vi "PWROpen.vi"(8 "error in (no error)":errorcluster {"code" format="%.0x"}, 11 "PWR In":refnum<visa-resource-name>) -> (0 "error out":errorcluster, 3 "PWR Out":refnum<visa-resource-name>, 5 "PWRID":u8)   [LabVIEW 2015]
uses:
  <instrlib>/Agilent N87XX Series/Agilent N87XX Series.lvlib
  <instrlib>/Agilent N6700 Series/Agilent N6700 Series.lvlib
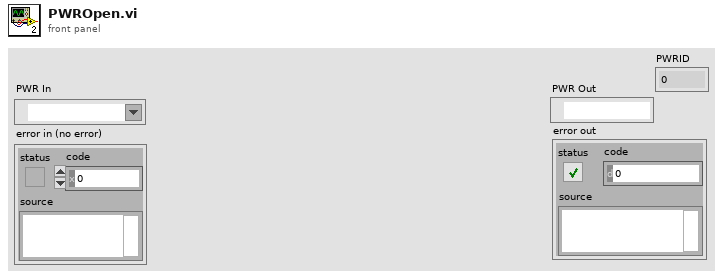
[diagram p1: front panel]
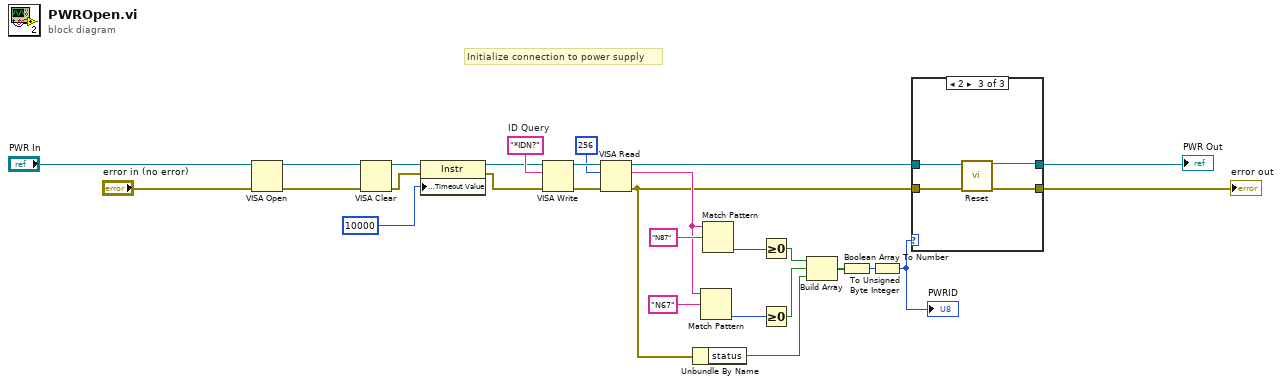
[diagram p0: block diagram]
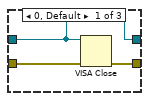
[diagram p2: hidden frame]
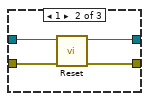
[diagram p3: hidden frame]
diagram:
  w24 = "*IDN?"  # ID Query
  # "Initialize connection to power supply"
  n1 = VISA Open(error in (no error)="error in (no error)", VISA resource name="PWR In") -> (VISA resource name=w21:refnum<visa-resource-name>, error out=w22:errorcluster)  [unwired: 3 in]
  n2 = VISA Clear(VISA resource name=w21, error in (no error)=w22) -> (VISA resource name out=w8:refnum<visa-resource-name>, error out=w7:errorcluster)
  n3 = property class="Instr"(reference=w8, error in=w7, "General Settings:Timeout Value"=u32 10000) -> (reference out=w6:refnum<visa-resource-name>, error out=w5:errorcluster)
  n4 = VISA Write(VISA resource name=w6, write buffer=w24, error in (no error)=w5) -> (VISA resource name out=w28:refnum<visa-resource-name>, error out=w27:errorcluster)  [unwired: 1 out]
  n5 = VISA Read(VISA resource name=w28, byte count=u32 256, error in (no error)=w27) -> (VISA resource name out=w13:refnum<visa-resource-name>, read buffer=w19:string, error out=w10:errorcluster)  [unwired: 1 out]
  n6 = Unbundle By Name(w10) -> ("status"=w9:bool)
  n7 = Match Pattern(string=w19, regular expression="N67") -> (offset past match=w17:i32)  [unwired: 1 in, 3 out]
  n8 = Match Pattern(string=w19, regular expression="N87") -> (offset past match=w23:i32)  [unwired: 1 in, 3 out]
  n9 = Greater Or Equal To 0?(x=w23) -> (x >= 0?=w16:bool)
  n10 = Greater Or Equal To 0?(x=w17) -> (x >= 0?=w15:bool)
  n11 = Build Array(w16, w15, w9) -> (w14:bool[])
  n12 = Boolean Array To Number(Boolean array=w14) -> (number=w3:u32)
  n13 = To Unsigned Byte Integer(number=w3) -> (unsigned 8bit integer=w2:u8)
  "PWRID" <- w2
  n14 = case shown="2" w2 {
    tunnel: w10 -> [w31 w34 w39]
    tunnel: w13 -> [w29 w35 w38]
    tunnel: [w29 w33 w37] -> w12
    tunnel: [w30 w32 w36] -> w11
    frame 0, Default {
      n15 = VISA Close(VISA resource name=w29, error in (no error)=w31) -> (error out=w30:errorcluster)
    }
    frame 1 {
      n16 = call <instrlib>:"Reset.vi"("error in (no error)"=w34, "VISA resource name"=w35) -> ("error out"=w32:errorcluster, "VISA resource name out"=w33:refnum<visa-resource-name>)  [unwired: 8 in]
    }
    frame 2 {
      n17 = call <instrlib>:"Reset.vi"("VISA resource name"=w38, "error in (no error)"=w39) -> ("VISA resource name out"=w37:refnum<visa-resource-name>, "error out"=w36:errorcluster)  [unwired: 12 in]
    }
  }
  "PWR Out" <- w12
  "error out" <- w11
